vi "ros2.vi"() -> ()   [LabVIEW 2015]
uses:
  <vilib>/Tufts CEEO ROS for LabVIEW Software/ROS/Code/Console/Servers/ServerSubs/TopicDef.ctl
  <vilib>/Tufts CEEO ROS for LabVIEW Software/ROS/Code/SubVIs/_ROSDirection.ctl
  <vilib>/Tufts CEEO ROS for LabVIEW Software/ROS/MessageBuilding/std_msgs/subs/boolScalar.vi
panel:
  out "msg out":string
  in  "Boolean":bool
  in  "node":string
  in  "Definitions":T1={"Topic"="/robot/head/command_head_nod", "Type"="std_msgs/Bool", "Action"=enum."Publisher", "Update (ms)"=1, "queue size"=1}
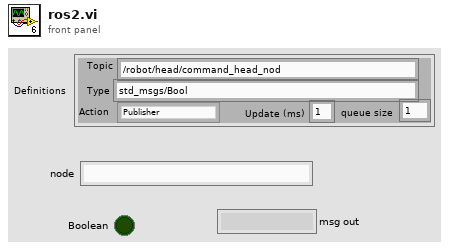
[diagram p1: front panel]
types:
  T1 = typedef "TopicDef.ctl" = cluster{"Topic":string, "Type":string, "Action":T2, "Update (ms)":u16, "queue size":u16}
  T2 = typedef "_ROSDirection.ctl" = enum16{"Node", "Publisher", "Subscriber", "ServiceClient", "ServiceProvider"}
  T3 = typedef "_ROSControl.ctl" = cluster{"topic port":u16, "Node":string, "topic":string, "type":string, "node port":u16, "error ":errorcluster, "Direction":T2, "Update (ms)":u16, "FIFO size":u16}
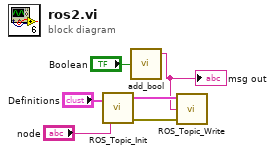
[diagram p0: block diagram]
diagram:
  n1 = call <vilib>:"ROS_Topic_Init.vi"("Definitions"="Definitions", "node"="node") -> ("ROS out"=w6:T3, "error out"=w5:errorcluster)  [unwired: 1 in]
  n2 = call-poly <vilib>:"add_bool.vi"("Boolean"="Boolean") -> ("msg out"=w2:string)  [unwired: 4 in]
  "msg out" <- w2
  n3 = call <vilib>:"ROS_Topic_Write.vi"("error in (no error)"=w5, "Msg in"=w2, "ROS in"=w6) -> ()  [unwired: 1 in, 2 out]
